vi "FPGA Main Default.vi"() -> ()   [LabVIEW 2015]
doc: "The myRIO v1.1 FPGA Shipping Personality. This personality contains support for:\n- 2 Analog Input Interrupt channel\n- 4 Digital Input Interrupt channel\n- 1 Timer\n- 1 Accelerometer\n- 1 Button\n- 4 LED\n- 10 Analog Input channels with 1 Sample\n- 6 Analog Output channels with 1 Sample\n- 40 Digital I/O channels with 1 Sample\n- 2 I2C channels\n- 4 Encoder channels\n- 6 PWM channels\n- 2 SPI channels"
uses:
  Sub VIs/Utilities/Start Boolean.ctl
  <vilib>/Platform/TimedLoop/XDataNode/timing_clust.ctl
  <vilib>/Platform/TimedLoop/XDataNode/nitl_modes.ctl
  <vilib>/Platform/TimedLoop/XDataNode/wakeup.ctl
  <vilib>/rvi/Emulation/niFpgaGetClockAttributes.vi
  <vilib>/rvi/Emulation/niFpgaSctlEmulationGetInTimedLoop.vi
  <vilib>/rvi/Emulation/niFpgaEmulationReportErrorSimple.vi
  <vilib>/rvi/eio/common/nirviEmuTemplateMethod_errors.vi
  <vilib>/rvi/Emulation/niFpgaCriticalErrorInLSC.vi
  <vilib>/rvi/Emulation/niFpgaProcessEmulError.vi
  <vilib>/eio/EIONode/EIONode.xnode
  <vilib>/Platform/TimedLoop/XDataNode/XDataNode.xnode
  <vilib>/Platform/TimedLoop/XDataNode/XDNodeRunTimeDep.lvlib
panel:
  out "DI.BTN":u8 format="%08b"
  out "DIO.B_3:0.IN 2":u8 format="%04b"
  out "ENC.3.STAT":u8 format="%08b"
  out "ENC.3.CNTR":u32
  in  "ENC.3.CNFG":u8 format="%08b"
  in  "DIO.B_3:0.OUT 2":u8 format="%04b"
  out "DIO.B_3:0.IN 1":u8 format="%04b"
  in  "DIO.B_3:0.OUT 1":u8 format="%04b"
  in  "AO.A_0.VAL":u16
  in  "AO.A_1.VAL":u16
  in  "AO.B_0.VAL":u16
  in  "AO.B_1.VAL":u16
  out "AI.B_3.VAL":u16
  out "AI.B_2.VAL":u16
  out "AI.B_1.VAL":u16
  out "AI.B_0.VAL":u16
  out "AI.A_3.VAL":u16
  out "AI.A_2.VAL":u16
  out "AI.A_1.VAL":u16
  out "AI.A_0.VAL":u16
  in  "ENC.2.CNFG":u8 format="%08b"
  in  "ENC.1.CNFG":u8 format="%08b"
  out "ENC.2.CNTR":u32
  out "ENC.1.CNTR":u32
  out "ENC.2.STAT":u8 format="%08b"
  out "ENC.1.STAT":u8 format="%08b"
  out "SYS.AI.RDY":bool
  out "SYS.RDY":bool
  out "AI.C_1.VAL":u16
  out "AI.C_0.VAL":u16
  in  "AO.C_0.VAL":u16
  in  "AO.C_1.VAL":u16
  in  "AO.SYS.GO":T1
  in  "DO.LED3:0":u8 format="%04b"
  out "AO.SYS.STAT":bool
  # "Connector B"
  # "Connector C"
  # "System"
  # "Onboard Devices"
  # "Connector A"
  # "Analog Input"
  # "Analog Output"
  # "Digital I/O"
  # "Encoders"
  # "Analog Input"
  # "Analog Output"
  # "Analog Input"
  # "Analog Output"
  # "Digital I/O"
  # "Encoders"
  # "Buttons & LEDs"
  # "Outputs"
  # "Input"
  # "Encoders Motor 1"
  # "Encoders Motor 3"
  # "IO Configuration"
  # "IO Configuration"
  # "Chn. A = DO11\nChn. B = DIO12"
  # "Chn. A = DO11\nChn. B = DIO12"
  # "IO Configuration"
  # "Bit 0 = Enable pin motor controller 1\nBit 1 = Direction pin motor controller 1\nBit 2 = Enable pin motor controller 2\nBit 3 = Direction pin motor ontroller 2"
  # "Bit 0 = Enable pin motor controller 3  \nBit 1 = Direction pin motor controller  3\nBit 2 = Enable tx modbus RS-485\nBit 3 = Reserve"
  # "Bit 0 = Reed switch links motor 3   \nBit 1 = Reed switch rechts motor 3\nBit 2 = Reserve \nBit 3 = Reserve"
  # "Bit 0 = Reed switch links motor 1   \nBit 1 = Reed switch rechts motor 1 \nBit 2 = Reed switch links motor 2 \nBit 3 = Reed switch rechts motor 2"
  # "Encoders Motor 2"
  # "Bit 0 = DIO4 \nBit 1 = DIO5\nBit 2 = DIO6\nBit 3 = DIO7"
  # "Bit 0 = DIO4 \nBit 1 = DIO5\nBit 2 = DIO6\nBit 3 = DIO7"
  # "Bit 0 = DIO0 \nBit 1 = DIO1\nBit 2 = DIO2\nBit 3 = DIO3"
  # "Bit 0 = DIO0 \nBit 1 = DIO1\nBit 2 = DIO2\nBit 3 = DIO3"
  # "Chn. A = DO13\nChn. B = DIO14"
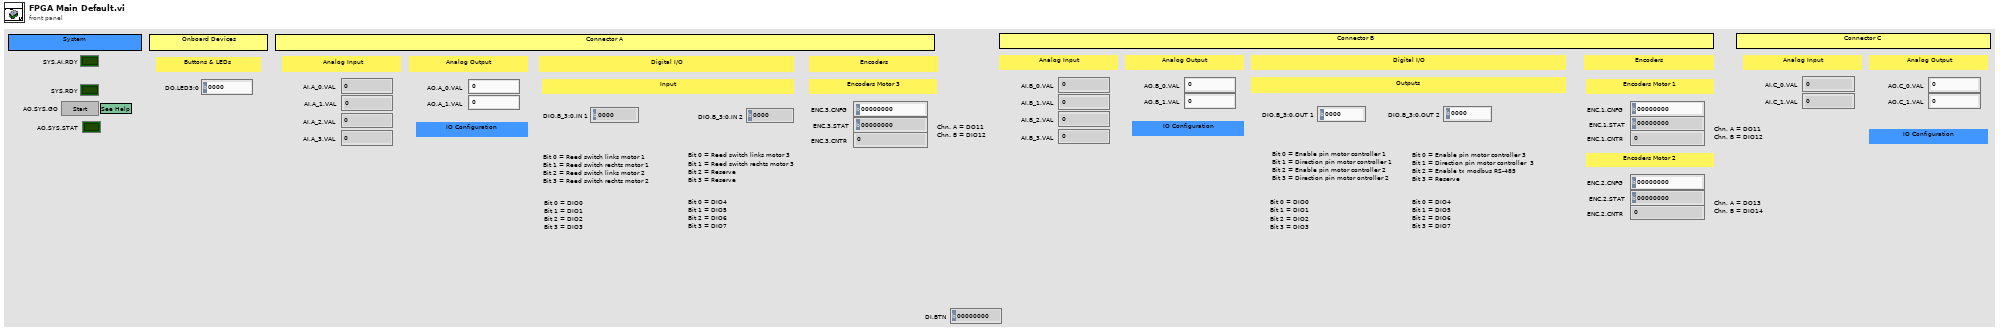
[diagram p1: front panel]
types:
  T1 = typedef "Start Boolean.ctl" = bool
  T2 = typedef "XDNodeRunTimeDep.lvlib/timing_clust.ctl" = cluster{"Expected End [f-1]":u64, "Actual End [f-1]":u64, "Finished Late? [f-1]":bool, "Expected End [i-1]":u64, "Actual End [i-1]":u64, "Finished Late? [i-1]":bool, "Expected Start [i]":u64, "Actual Start [i]":u64, "Expected Start [f]":u64, "Actual Start [f]":u64, "Source Name":string, "Structure Name":string, "Period":i64, "Deadline":i64, "Offset":i64, "Start":i64, "Priority":i32, "Timeout":i32, "Mode":T3, "Wakeup Reason":T4, "Error":errorcluster, "Source Type":string, "Secondary Source Type":string, "Global End Time":u64, "Global Start Time":u64, "Frame Duration":u64, "Iteration Duration":u64, "Assigned CPU":i32, "I/O Scan Engine Mode":u32}
  T3 = typedef "XDNodeRunTimeDep.lvlib/nitl_modes.ctl" = enum32{"No Change", "Process missed periods, maintain original phase", "Discard missed periods, maintain original phase", "Process missed periods, ignore original phase", "Discard missed periods, ignore original phase"}
  T4 = typedef "XDNodeRunTimeDep.lvlib/wakeup.ctl" = enum32{"Normal", "Aborted", "Asynchronous wakeup", "Timing source error", "Timed loop error", "Timeout"}
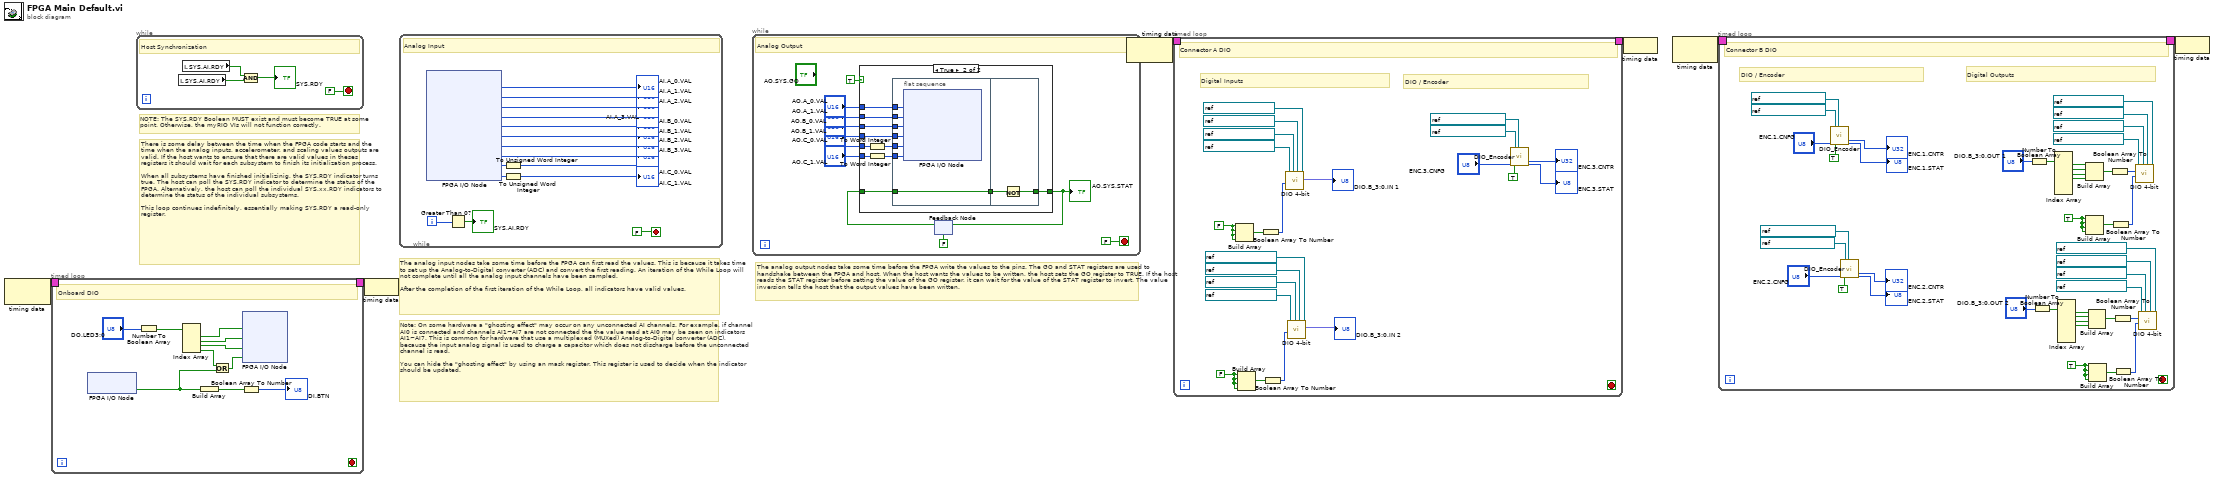
[diagram p0: block diagram]
diagram:
  # "The analog output nodes take some time before the FPGA write the values to the pins. The GO and STAT registers are used to handshake between the FPGA and host. When the host wants the values to be written, the host sets the GO register to TRUE. If the host reads the STAT register before setting the value of the GO register, it can wait for the value of the STAT register to invert. The value inversion tells the host that the output values have been written."
  # "The analog input nodes take some time before the FPGA can first read the values. This is because it takes time to set up the Analog-to-Digital converter (ADC) and convert the first reading. An iteration of the While Loop will not complete until all the analog input channels have been sampled.\n\nAfter the completion of the first iteration of the While Loop, all indicators have valid values."
  # "Note: On some hardware a \"ghosting effect\" may occur on any unconnected AI channels. For example, if channel AI0 is connected and channels AI1~AI7 are not connected the the value read at AI0 may be seen on indicators AI1~AI7. This is common for hardware that use a multiplexed (MUXed) Analog-to-Digital converter (ADC), because the input analog signal is used to charge a capacitor which does not discharge before the unconnected channel is read.\n\nYou can hide the \"ghosting effect\" by using an mask register. This register is used to decide when the indicator should be updated."
  # "NOTE: The SYS.RDY Boolean MUST exist and must become TRUE at some point. Otherwise, the myRIO VIs will not function correctly."
  # "There is some delay between the time when the FPGA code starts and the time when the analog inputs, accelerometer, and scaling values outputs are valid. If the host wants to ensure that there are valid values in theses registers it should wait for each subsystem to finish its initialization process. \n\nWhen all subsystems have finished initializinig, the SYS.RDY indicator turns true. The host can poll the SYS.RDY indicator to determine the status of the FPGA. Alternatively, the host can poll the individual SYS.xx.RDY indicators to determine the status of the individual subsystems.\n\nThis loop continues indefinitely, essentially making SYS.RDY a read-only register."
  n1 = node-c288() -> (w4:T2)  [unwired: 1 in]
  n2 = timed-loop {
    timing: w4 -> [_]
    timing-out: [_] -> w3
    stop <- _ stop-if-true
    # "Onboard DIO"
    n3 = xnode "FPGA I/O Node"() -> ("Button0"=w8:bool)  [unwired: 1 in, 1 out]
    n4 = Number To Boolean Array(number="DO.LED3:0") -> (Boolean array=w15:bool[])
    n5 = Index Array(array=w15) -> (element #1=w14:bool, element #2=w13:bool, element #3=w12:bool, element #4=w9:bool)  [unwired: 4 in]
    n6 = Build Array(w8) -> (w11:bool[])
    n7 = Or(x=w9, y=w8) -> (x .or. y?=w7:bool)
    n8 = xnode "FPGA I/O Node"("LED0"=w14, "LED1"=w13, "LED2"=w12, "LED3"=w7) -> ()  [unwired: 4 in, 4 out]
    n9 = Boolean Array To Number(Boolean array=w11) -> (number=→"DI.BTN":u8)
  }
  n10 = while {
    stop <- FALSE stop-if-true
    # "Host Synchronization"
    n11 = local read "SYS.AI.RDY"() -> (w20:bool)
    n12 = local read "SYS.AI.RDY"() -> (w22:bool)
    n13 = Compound Arithmetic op=AND(w22, w20) -> (→"SYS.RDY":bool)
  }
  n14 = node-c288(w3) -> ()
  n15 = while {
    i -> [w34]
    stop <- FALSE stop-if-true
    # "Analog Input"
    n16 = xnode "FPGA I/O Node"() -> ("ConnectorA/AI0"=→"AI.A_0.VAL":u16, "ConnectorA/AI1"=→"AI.A_1.VAL":u16, "ConnectorA/AI2"=→"AI.A_2.VAL":u16, "ConnectorA/AI3"=→"AI.A_3.VAL":u16, "ConnectorB/AI0"=→"AI.B_0.VAL":u16, "ConnectorB/AI1"=→"AI.B_1.VAL":u16, "ConnectorB/AI2"=→"AI.B_2.VAL":u16, "ConnectorB/AI3"=→"AI.B_3.VAL":u16, "ConnectorC/AI0"=w28:i16, "ConnectorC/AI1"=w27:i16)  [unwired: 10 in, 10 out]
    n17 = Greater Than 0?(x=w34) -> (x > 0?=→"SYS.AI.RDY":bool)
    n18 = To Unsigned Word Integer(number=w28) -> (unsigned 16bit integer=→"AI.C_0.VAL":u16)
    n19 = To Unsigned Word Integer(number=w27) -> (unsigned 16bit integer=→"AI.C_1.VAL":u16)
  }
  n20 = while {
    stop <- FALSE stop-if-true
    # "Analog Output"
    n21 = feedback #1(FALSE) -> (w40:bool)
    n22 = case shown="True" TRUE {
      tunnel: "AO.C_0.VAL" -> [_ w56]
      tunnel: "AO.C_1.VAL" -> [_ w55]
      tunnel: "AO.A_0.VAL" -> [_ w60]
      tunnel: "AO.A_1.VAL" -> [_ w59]
      tunnel: "AO.B_0.VAL" -> [_ w58]
      tunnel: "AO.B_1.VAL" -> [_ w57]
      tunnel: w40 -> [w49 w52]
      tunnel: [w49 w50] -> w39
      frame False {
      }
      frame True {
        n23 = To Word Integer(number=w56) -> (16bit integer=w54:i16)
        n24 = To Word Integer(number=w55) -> (16bit integer=w53:i16)
        n25 = flat-sequence {
          tunnel: w60 -> [w67]
          tunnel: w59 -> [w66]
          tunnel: w58 -> [w65]
          tunnel: w57 -> [w64]
          tunnel: w54 -> [w63]
          tunnel: w53 -> [w62]
          tunnel: w52 -> [w61]
          tunnel: [w61] -> w51
          tunnel: w51 -> [w69]
          tunnel: [w68] -> w50
          frame #0 {
            n26 = xnode "FPGA I/O Node"("ConnectorA/AO0"=w67, "ConnectorA/AO1"=w66, "ConnectorB/AO0"=w65, "ConnectorB/AO1"=w64, "ConnectorC/AO0"=w63, "ConnectorC/AO1"=w62) -> ()  [unwired: 6 in, 6 out]
          }
          frame #1 {
            n27 = Not(x=w69) -> (.not. x?=w68:bool)
          }
        }
      }
    }
    "AO.SYS.STAT" <- w39
    n28 = feedback-in #1(w39) -> ()
  }
  n29 = node-c288() -> (w2:T2)  [unwired: 1 in]
  n30 = timed-loop {
    timing: w2 -> [_]
    timing-out: [_] -> w1
    stop <- _ stop-if-true
    w82 = FALSE
    w90 = FALSE
    # "DIO / Encoder"
    # "Digital Inputs"
    # "Connector A DIO"
    n31 = Build Array(w90, w90, w90, w90) -> (w89:bool[])
    n32 = Build Array(w82, w82, w82, w82) -> (w81:bool[])
    n33 = Boolean Array To Number(Boolean array=w89) -> (number=w91:u8)
    n34 = Boolean Array To Number(Boolean array=w81) -> (number=w83:u8)
    n35 = call "DIO 4-bit.vi"("DIO0 Refnum"=refnum<k21> "ConnectorA/DIO0", "DIO1 Refnum"=refnum<k21> "ConnectorA/DIO1", "DIO2 Refnum"=refnum<k21> "ConnectorA/DIO2", "DIR 3:0"=w91, "DIO3 Refnum"=refnum<k21> "ConnectorA/DIO3") -> ("IN 3:0"=→"DIO.B_3:0.IN 1":fxp<+,4,4>)  [unwired: 6 in]
    n36 = call "DIO 4-bit.vi"("DIO0 Refnum"=refnum<k21> "ConnectorA/DIO4", "DIO1 Refnum"=refnum<k21> "ConnectorA/DIO5", "DIO2 Refnum"=refnum<k21> "ConnectorA/DIO6", "DIR 3:0"=w83, "DIO3 Refnum"=refnum<k21> "ConnectorA/DIO7") -> ("IN 3:0"=→"DIO.B_3:0.IN 2":fxp<+,4,4>)  [unwired: 6 in]
    n37 = call "DIO_Encoder.vi"("QE.CNFG"="ENC.3.CNFG", "DIO.1/QE.B"=refnum<k21> "ConnectorA/DIO12", "SELECT"=TRUE, "DIO.0/QE.A"=refnum<k21> "ConnectorA/DIO11") -> ("QE.CNTR"=→"ENC.3.CNTR":u32, "QE.STAT"=→"ENC.3.STAT":u8)  [unwired: 13 in, 1 out]
  }
  n38 = node-c288(w1) -> ()
  n39 = node-c288() -> (w6:T2)  [unwired: 1 in]
  n40 = timed-loop {
    timing: w6 -> [_]
    timing-out: [_] -> w5
    stop <- _ stop-if-true
    w105 = TRUE
    w120 = TRUE
    # "DIO / Encoder"
    # "Digital Outputs"
    # "Connector B DIO"
    n41 = call "DIO_Encoder.vi"("QE.CNFG"="ENC.1.CNFG", "DIO.1/QE.B"=refnum<k21> "ConnectorB/DIO12", "SELECT"=TRUE, "DIO.0/QE.A"=refnum<k21> "ConnectorB/DIO11") -> ("QE.CNTR"=→"ENC.1.CNTR":u32, "QE.STAT"=→"ENC.1.STAT":u8)  [unwired: 13 in, 1 out]
    n42 = call "DIO_Encoder.vi"("QE.CNFG"="ENC.2.CNFG", "DIO.1/QE.B"=refnum<k21> "ConnectorB/DIO14", "SELECT"=TRUE, "DIO.0/QE.A"=refnum<k21> "ConnectorB/DIO13") -> ("QE.CNTR"=→"ENC.2.CNTR":u32, "QE.STAT"=→"ENC.2.STAT":u8)  [unwired: 13 in, 1 out]
    n43 = Number To Boolean Array(number="DIO.B_3:0.OUT 1") -> (Boolean array=w128:bool[])
    n44 = Number To Boolean Array(number="DIO.B_3:0.OUT 2") -> (Boolean array=w113:bool[])
    n45 = Index Array(array=w128) -> (element #1=w127:bool, element #2=w126:bool, element #3=w125:bool, element #4=w124:bool)  [unwired: 7 in, 3 out]
    n46 = Index Array(array=w113) -> (element #1=w112:bool, element #2=w111:bool, element #3=w110:bool, element #4=w109:bool)  [unwired: 7 in, 3 out]
    n47 = Build Array(w127, w126, w125, w124) -> (w123:bool[])
    n48 = Build Array(w120, w120, w120, w120) -> (w119:bool[])
    n49 = Build Array(w112, w111, w110, w109) -> (w108:bool[])
    n50 = Build Array(w105, w105, w105, w105) -> (w104:bool[])
    n51 = Boolean Array To Number(Boolean array=w123) -> (number=w122:u8)
    n52 = Boolean Array To Number(Boolean array=w119) -> (number=w121:u8)
    n53 = Boolean Array To Number(Boolean array=w108) -> (number=w107:u8)
    n54 = Boolean Array To Number(Boolean array=w104) -> (number=w106:u8)
    n55 = call "DIO 4-bit.vi"("DIO0 Refnum"=refnum<k21> "ConnectorB/DIO0", "DIO1 Refnum"=refnum<k21> "ConnectorB/DIO1", "DIO2 Refnum"=refnum<k21> "ConnectorB/DIO2", "DIR 3:0"=w121, "OUT 3:0"=w122, "DIO3 Refnum"=refnum<k21> "ConnectorB/DIO3") -> ()  [unwired: 5 in, 1 out]
    n56 = call "DIO 4-bit.vi"("DIO0 Refnum"=refnum<k21> "ConnectorB/DIO4", "DIO1 Refnum"=refnum<k21> "ConnectorB/DIO5", "DIO2 Refnum"=refnum<k21> "ConnectorB/DIO8", "DIR 3:0"=w106, "OUT 3:0"=w107, "DIO3 Refnum"=refnum<k21> "ConnectorB/DIO9") -> ()  [unwired: 5 in, 1 out]
  }
  n57 = node-c288(w5) -> ()
